vi "Cambio Long PEM.vi"(2 "error in":errorcluster, 3 "Long de Onda":dbl, 4 "VISA Refnum in":refnum<visa-resource-name>) -> (0 "error out":errorcluster, 1 "VISA Refnum out":refnum<visa-resource-name>)   [LabVIEW 2016]
panel:
  out "Frecuency":dbl format="%_5f"
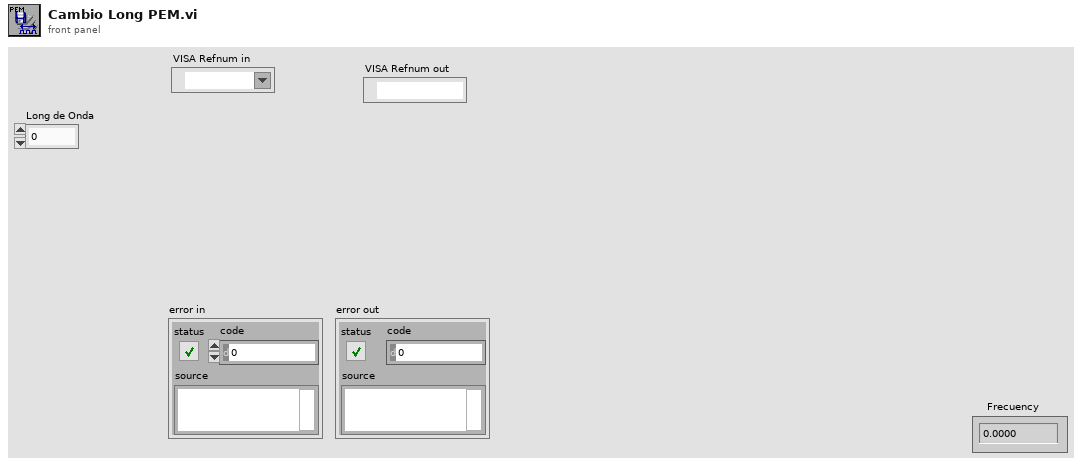
[diagram p1: front panel]
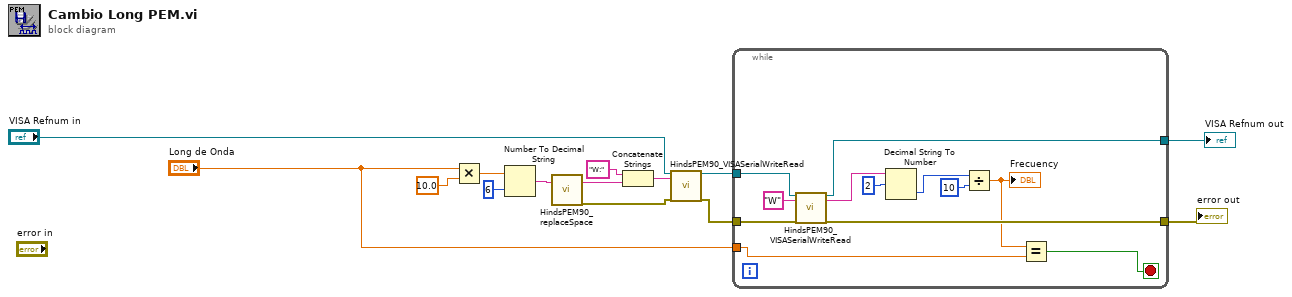
[diagram p0: block diagram]
diagram:
  n1 = Multiply(x="Long de Onda", y=10.0) -> (x*y=w9:dbl)
  n2 = Number To Decimal String(number=w9, width (-)=i16 6) -> (decimal integer string=w8:string)
  n3 = call "HindsPEM90_replaceSpace.vi"("Sting In"=w8) -> ("String Out"=w7:string, "error out"=w14:errorcluster)  [unwired: 17 in]
  n4 = Concatenate Strings("W:" ("Substring"), w7) -> (w12:string)
  n5 = call "HindsPEM90_VISASerialWriteRead.vi"("VISA refnum in"="VISA Refnum in", "write"=w12, "error in (no error)"=w14) -> ("VISA refnum out"=w5:refnum<visa-resource-name>, "error out"=w4:errorcluster)  [unwired: 14 in, 1 out]
  n6 = while {
    tunnel: w5 -> [w21]
    tunnel: w4 -> [w20]
    tunnel: [w19] -> w3
    tunnel: [w18] -> w2
    tunnel: "Long de Onda" -> [w16]
    stop <- w15 stop-if-true
    n7 = call "HindsPEM90_VISASerialWriteRead.vi"("VISA refnum in"=w21, "write"="W" ("Substring"), "error in (no error)"=w20) -> ("VISA refnum out"=w19:refnum<visa-resource-name>, "read buffer"=w25:string, "error out"=w18:errorcluster)  [unwired: 14 in]
    n8 = Decimal String To Number(string=w25, offset=2) -> (number=w23:i32)  [unwired: 1 in, 1 out]
    n9 = Divide(x=w23, y=10) -> (x/y=w17:dbl)
    "Frecuency" <- w17
    n10 = Equal?(x=w17, y=w16) -> (x = y?=w15:bool)
  }
  "error out" <- w2
  "VISA Refnum out" <- w3
